vi "overlay line.vi"(0 "垂直方向第一点":cluster{"第二点x值，y=1023":dbl, dbl}, 2 "垂直方向第二点":cluster{"第二点x值，y=1023":dbl, dbl}, 3 "水平方向第一点":cluster{"第二点x值，y=1023":dbl, dbl}, 5 "水平方向第二点":cluster{"第二点x值，y=1023":dbl, dbl}, 6 "触发":bool, 7 "error in":errorcluster, 8 "Image in":T1, 9 "Color":u32(colorbox)=16711680) -> (14 "Image Out 2":T1, 19 "error out":errorcluster)   [LabVIEW 2015]
uses:
  <vilib>/vision/Image Controls.llb/IMAQ Image.ctl
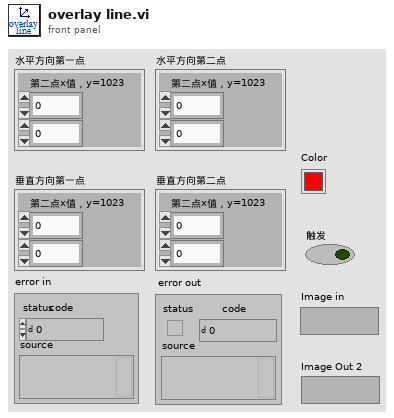
[diagram p1: front panel]
types:
  T1 = typedef "IMAQ Image.ctl" = refnum<image>
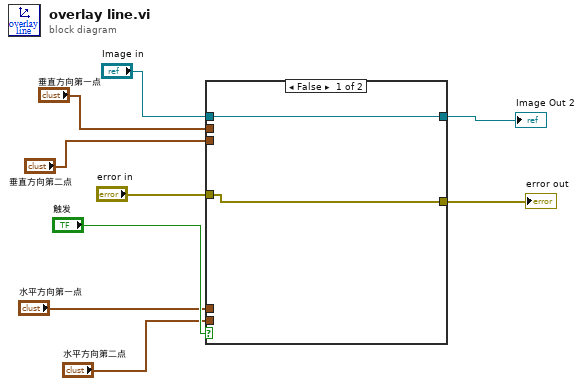
[diagram p0: block diagram]
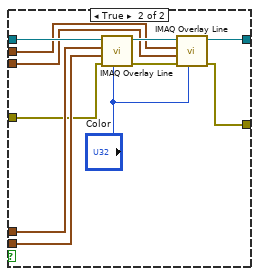
[diagram p2: hidden frame]
diagram:
  n1 = case shown="False" "触发" {
    tunnel: [w11 w20] -> w3
    tunnel: "Image in" -> [w11 w19]
    tunnel: "水平方向第一点" -> [_ w18]
    tunnel: "水平方向第二点" -> [_ w17]
    tunnel: "垂直方向第一点" -> [_ w16]
    tunnel: "垂直方向第二点" -> [_ w15]
    tunnel: "error in" -> [w10 w13]
    tunnel: [w10 w12] -> w1
    frame False {
    }
    frame True {
      n2 = call "IMAQ Overlay Line"("Color"="Color", "error in (no error)"=w13, "End Point"=w17, "Start Point"=w18, "Image"=w19) -> ("error out"=w22:errorcluster, "Image Out"=w21:T1)  [unwired: 5 in]
      n3 = call "IMAQ Overlay Line"("Color"="Color", "error in (no error)"=w22, "End Point"=w15, "Start Point"=w16, "Image"=w21) -> ("error out"=w12:errorcluster, "Image Out"=w20:T1)  [unwired: 5 in]
    }
  }
  "Image Out 2" <- w3
  "error out" <- w1
